vi "Read JSON File (LV).vi"(7 "Default Value":variant, 8 "error in (no error)":errorcluster, 11 "file path (use dialog)":path) -> (0 "error out":errorcluster, 3 "Value":variant)   [LabVIEW 2015, in "JSON.lvlib"]
uses:
  JSON.lvlib
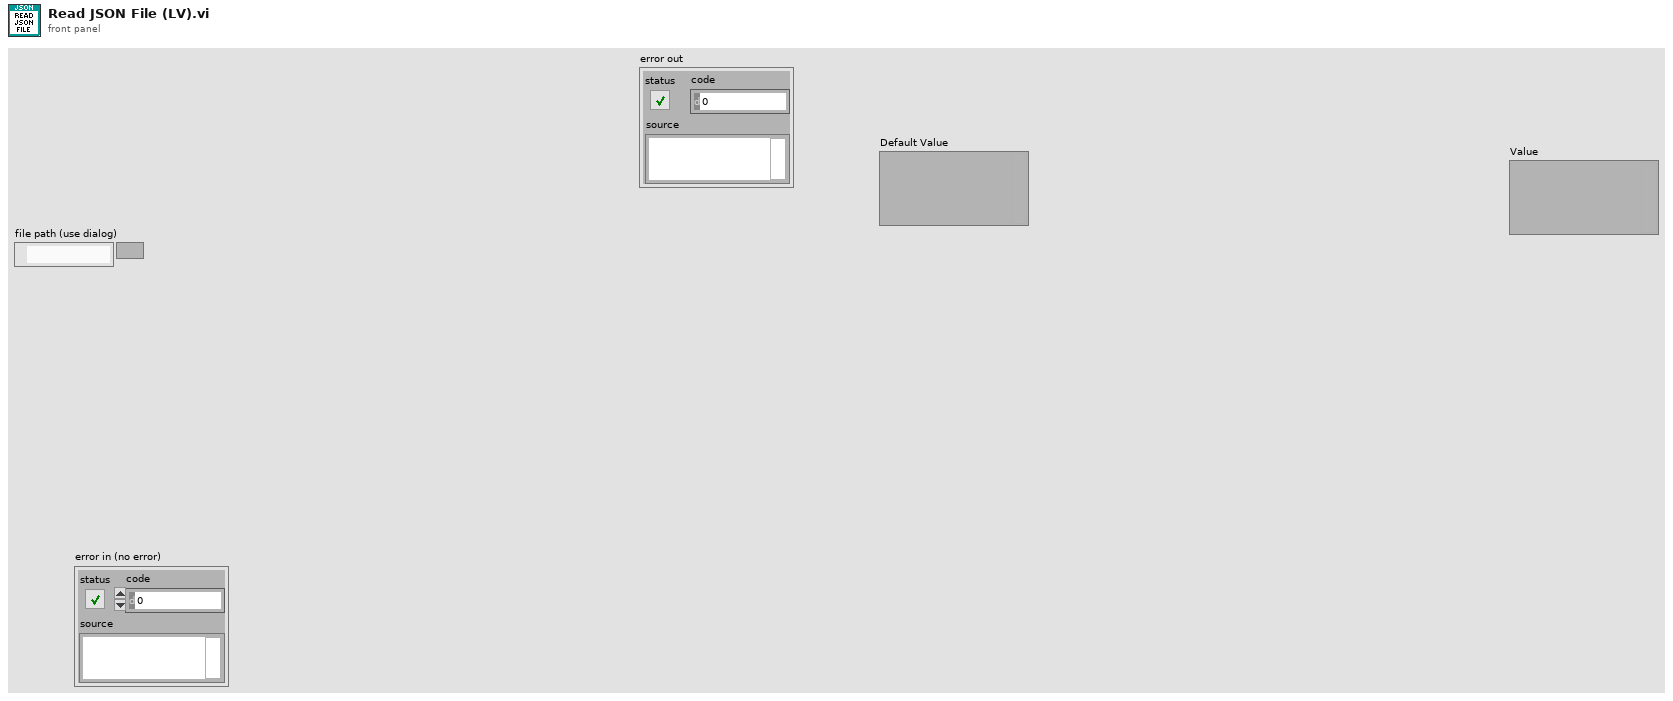
[diagram p1: front panel]
types:
  T1 = enum16{"open", "replace", "create", "open or create", "replace or create", "replace or create with confirmation"}
  T2 = typedef "JSON.lvlib/JSON Value.ctl" = cluster{"\\type":enum16{"Object", "Array", "String", "Number", "Boolean", "Null"}, "ÿýÿýÿýÿýÿýÿþÿýÿýÿý&LV-JSON.lvlib:JSON Name-Value Pair.ctlÿýÿýÿýÿýÿýÿþÿýÿýÿýLV-JSON.lvlib:JSON Value.ctl":variant}
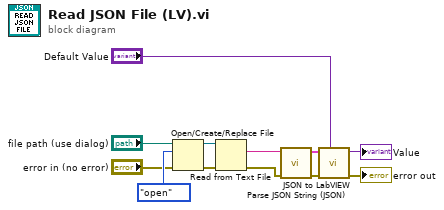
[diagram p0: block diagram]
diagram:
  n1 = Open/Create/Replace File(file path (use dialog)="file path (use dialog)", error in="error in (no error)", operation (0:open)=T1."open") -> (refnum out=w9:refnum<file>, error out=w10:errorcluster)  [unwired: 3 in, 1 out]
  n2 = Read from Text File(file (use dialog)=w9, error in=w10) -> (text=w7:string, error out=w1:errorcluster)  [unwired: 2 in, 2 out]
  n3 = call "Parse JSON String (JSON).vi"("error in (no error)"=w1, "String"=w7) -> ("error out"=w3:errorcluster, "Value"=w5:T2)  [unwired: 8 in]
  n4 = call "JSON to LabVIEW.vi"("Default Value"="Default Value", "error in (no error)"=w3, "JSON Value"=w5) -> ("error out"=→"error out":errorcluster, "LV Value"=→"Value":variant)  [unwired: 7 in]
